vi "Add Icon to Title & Description.vi"(9 "Background Color":u32(colorbox), 10 "Title & Description":picture, 11 "Icon":picture) -> (3 "Icon + Title & Description":picture)   [LabVIEW 2016, in "MetaDataObj.lvclass"]
uses:
  <resource>/dialog/NewProjectWizard/MetaDataObj/MetaDataObj.lvclass
  <vilib>/Utility/miscctls.llb/LVBoundsTypeDef.ctl
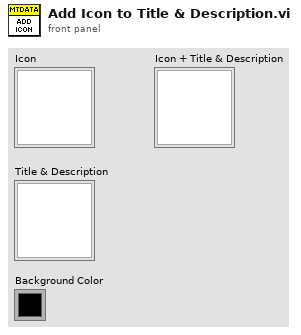
[diagram p1: front panel]
types:
  T1 = typedef "LVBoundsTypeDef.ctl" = cluster{"Width":u32, "Height":u32}
  T2 = typedef "imagedata.ctl" = cluster{"image type":i32, "image depth":i32, "image":u8[], "mask":u8[], "colors":u32[], "Rectangle":cluster{"left":i16, "top":i16, "right":i16, "bottom":i16}}
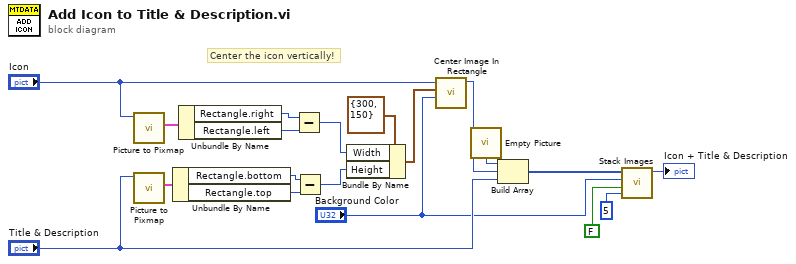
[diagram p0: block diagram]
diagram:
  # "Center the icon vertically!"
  n1 = call <vilib>:"Picture to Pixmap.vi"("picture"="Icon") -> ("image data"=w12:T2)  [unwired: 9 in, 1 out]
  n2 = call <vilib>:"Picture to Pixmap.vi"("picture"="Title & Description") -> ("image data"=w15:T2)  [unwired: 9 in, 1 out]
  n3 = Unbundle By Name(w15) -> ("Rectangle.bottom"=w14:i16, "Rectangle.top"=w4:i16)
  n4 = Unbundle By Name(w12) -> ("Rectangle.right"=w10:i16, "Rectangle.left"=w11:i16)
  n5 = Subtract(x=w10, y=w11) -> (x-y=w7:i16)
  n6 = Subtract(x=w14, y=w4) -> (x-y=w8:i16)
  n7 = Bundle By Name(cluster=T1 {"Width"=300, "Height"=150} ("Rectangle"), "Width"=w7, "Height"=w8) -> (w6:T1)
  n8 = call <resource>:"Center Image In Rectangle.vi"("Background Color"="Background Color", "Rectangle"=w6, "Picture In"="Icon") -> ("Picture Out (Centered)"=w5:picture)  [unwired: 8 in]
  n9 = call "Empty Picture"() -> ("empty picture"=w1:picture)
  n10 = Build Array(w1, w5, "Title & Description") -> (w17:picture[])
  n11 = call <resource>:"Stack Images.vi"("Padding"=u8 5, "Vertical?"=FALSE, "BG Color"="Background Color", "Array"=w17) -> ("empty picture"=→"Icon + Title & Description":picture)  [unwired: 7 in]
